vi "Control- StepMotor(SubVI).vi"(7 "Frequency (Hz)":u32=200, 8 "error in (no error)":errorcluster, 9 "LINX Resource in":T1={"IO"=enum."Remote", "Interface"=enum."Serial", "LINX Device Config"={"Interface"=enum."Serial", "COM Port"="COM12", "TCP Configuration"={"IP Address"="", "Port"=0}, "Device Family"=2, "Device ID"=5, "Device Name"="Arduino Nano 328\u0000", "TCP Ref"=refnum, "Channels"={"DI"=[0, 1, 2, 3, 4, 5, 6, 7, 8, 9, 10, 11, 12, 13], "DO"=[0, 1, 2, 3, 4, 5, 6, 7, 8, 9, 10, 11, 12, 13], "AI"=[0, 1, 2, 3, 4, 5, 6, 7], "AO"=[], "PWM"=[3, 5, 6, 9, 10, 11], "QE"=[], "UART"=[0], "I2C 2"=[0], "SPI"=[0], "CAN"=[], "Servo"=[0, 1, 2, 3, 4, 5, 6, 7, 8, 9, 10, 11, 12, 13], "AI Ref (V)"=5.0, "AI Resolution (Bits)"=0, "AO Ref (V)"=0.0, "AO Resolution (Bits)"=0}}}, 10 "DIR pin":u8=3, 11 "Pulse pin":u8=4) -> (0 "error out":errorcluster, 3 "LINX Resource out":T1={"IO"=enum."Remote", "Interface"=enum."Serial", "LINX Device Config"={"Interface"=enum."Serial", "COM Port"="COM12", "TCP Configuration"={"IP Address"="", "Port"=0}, "Device Family"=2, "Device ID"=5, "Device Name"="Arduino Nano 328\u0000", "TCP Ref"=refnum, "Channels"={"DI"=[0, 1, 2, 3, 4, 5, 6, 7, 8, 9, 10, 11, 12, 13], "DO"=[0, 1, 2, 3, 4, 5, 6, 7, 8, 9, 10, 11, 12, 13], "AI"=[0, 1, 2, 3, 4, 5, 6, 7], "AO"=[], "PWM"=[3, 5, 6, 9, 10, 11], "QE"=[], "UART"=[0], "I2C 2"=[0], "SPI"=[0], "CAN"=[], "Servo"=[0, 1, 2, 3, 4, 5, 6, 7, 8, 9, 10, 11, 12, 13], "AI Ref (V)"=5.0, "AI Resolution (Bits)"=0, "AO Ref (V)"=0.0, "AO Resolution (Bits)"=0}}})   [LabVIEW 2015]
uses:
  <vilib>/MakerHub/LINX/Private/Type Defs/LINX Ref.ctl
  <vilib>/MakerHub/LINX/Private/Type Defs/Platform.ctl
  <vilib>/MakerHub/LINX/Private/Type Defs/Interface.ctl
  <vilib>/MakerHub/LINX/Private/Device/Type Defs/LINX Device Config.ctl
  <vilib>/MakerHub/LINX/Private/Device/Type Defs/TCP Config.ctl
  <vilib>/MakerHub/LINX/Private/Device/Type Defs/Channels.ctl
  <vilib>/MakerHub/LINX/Public/Peripherals/Digital/Digital Write 1 Chan.vi
  <vilib>/MakerHub/LINX/Public/Peripherals/Digital/Digital Write N Chans.vi
  <vilib>/MakerHub/LINX/Private/Local IO/LinxDigitalWrite.vi
  <vilib>/MakerHub/LINX/Public/Utilities/Check Channel.vi
  <vilib>/MakerHub/LINX/Private/Utilties/Generate Error.vi
  <vilib>/MakerHub/LINX/LMH-LINX.lvlib
  <vilib>/MakerHub/LINX/Private/Device/Device.lvlib
panel:
  in  "Enable pin":u8=2
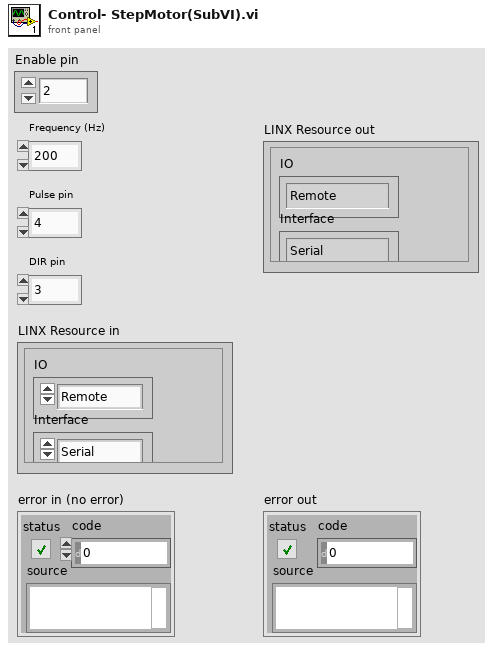
[diagram p1: front panel]
types:
  T1 = typedef "LMH-LINX.lvlib/LINX Ref.ctl" = cluster{"IO":T2, "Interface":T3, "LINX Device Config":T4}
  T2 = typedef "LMH-LINX.lvlib/Platform.ctl" = enum16{"Remote", "Local"}
  T3 = typedef "LMH-LINX.lvlib/Interface.ctl" = enum16{"Serial", "TCP"}
  T4 = typedef "LMH-LINX.lvlib/Device.lvlib/LINX Device Config.ctl" = cluster{"Interface":T3, "COM Port":refnum<visa-resource-name>, "TCP Configuration":T5, "Device Family":u8, "Device ID":u8, "Device Name":string, "TCP Ref":refnum<k5>, "Channels":T6}
  T5 = typedef "LMH-LINX.lvlib/Device.lvlib/TCP Config.ctl" = cluster{"IP Address":string, "Port":u16}
  T6 = typedef "LMH-LINX.lvlib/Channels.ctl" = cluster{"DI":u8[], "DO":u8[], "AI":u8[], "AO":u8[], "PWM":u8[], "QE":u8[], "UART":u8[], "I2C 2":u8[], "SPI":u8[], "CAN":u8[], "Servo":u8[], "AI Ref (V)":dbl, "AI Resolution (Bits)":u8, "AO Ref (V)":dbl, "AO Resolution (Bits)":u8}
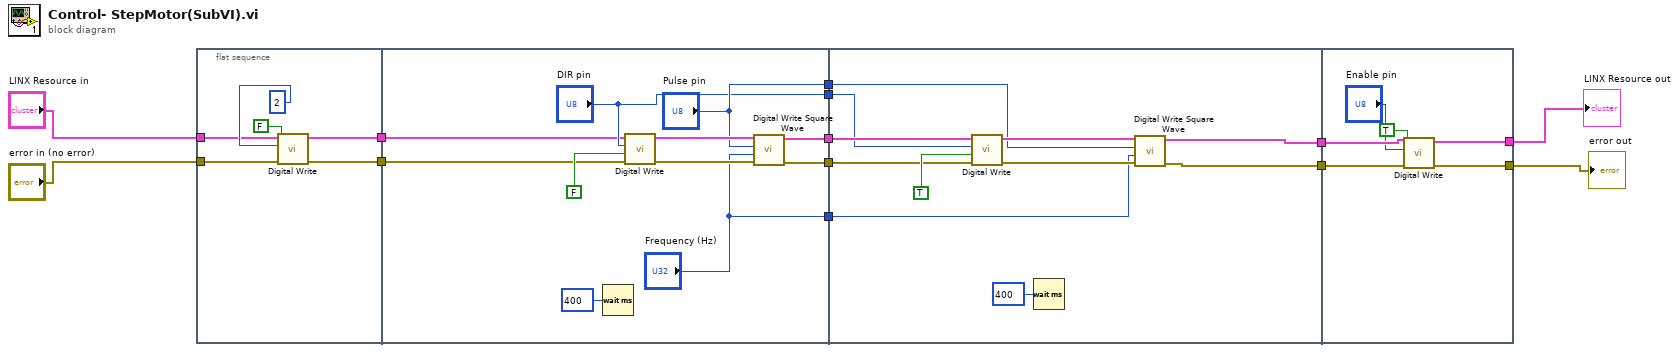
[diagram p0: block diagram]
diagram:
  n1 = flat-sequence {
    tunnel: "error in (no error)" -> [w16]
    tunnel: "LINX Resource in" -> [w17]
    tunnel: [w15] -> w2
    tunnel: [w14] -> w1
    tunnel: [w27] -> w13
    tunnel: [w26] -> w12
    tunnel: ["Frequency (Hz)"] -> w11
    tunnel: ["Pulse pin"] -> w10
    tunnel: ["DIR pin"] -> w9
    tunnel: w2 -> [w21]
    tunnel: w1 -> [w20]
    tunnel: w13 -> [w38]
    tunnel: w12 -> [w37]
    tunnel: w11 -> [w36]
    tunnel: w10 -> [w35]
    tunnel: w9 -> [w34]
    tunnel: [w32] -> w6
    tunnel: [w31] -> w5
    tunnel: w6 -> [w46]
    tunnel: w5 -> [w45]
    tunnel: [w44] -> w4
    tunnel: [w43] -> w3
    frame #0 {
      n2 = call-poly <vilib>:"Digital Write.vi"("Error In"=w16, "Output Value"=FALSE, "DO Channel"=u8 2, "LINX Resource"=w17) -> ("Error Out"=w14:errorcluster, "LINX Resource"=w15:T1)  [unwired: 6 in]
    }
    frame #1 {
      n3 = Wait (ms)(milliseconds to wait=u32 400) -> ()  [unwired: 1 out]
      n4 = call-poly <vilib>:"Digital Write.vi"("Error In"=w20, "Output Value"=FALSE, "DO Channel"="DIR pin", "LINX Resource"=w21) -> ("Error Out"=w29:errorcluster, "LINX Resource"=w30:T1)  [unwired: 6 in]
      n5 = call <vilib>:"Digital Write Square Wave.vi"("Error In"=w29, "Frequency (Hz)"="Frequency (Hz)", "Channel"="Pulse pin", "LINX Resource"=w30) -> ("Error Out"=w26:errorcluster, "LINX Resource"=w27:T1)  [unwired: 6 in]
    }
    frame #2 {
      n6 = call-poly <vilib>:"Digital Write.vi"("Error In"=w37, "Output Value"=TRUE, "DO Channel"=w34, "LINX Resource"=w38) -> ("Error Out"=w40:errorcluster, "LINX Resource"=w41:T1)  [unwired: 6 in]
      n7 = Wait (ms)(milliseconds to wait=u32 400) -> ()  [unwired: 1 out]
      n8 = call <vilib>:"Digital Write Square Wave.vi"("Error In"=w40, "Frequency (Hz)"=w36, "Channel"=w35, "LINX Resource"=w41) -> ("Error Out"=w31:errorcluster, "LINX Resource"=w32:T1)  [unwired: 6 in]
    }
    frame #3 {
      n9 = call-poly <vilib>:"Digital Write.vi"("Error In"=w45, "Output Value"=TRUE, "DO Channel"="Enable pin", "LINX Resource"=w46) -> ("Error Out"=w43:errorcluster, "LINX Resource"=w44:T1)  [unwired: 6 in]
    }
  }
  "error out" <- w3
  "LINX Resource out" <- w4
